vi "AES Encryption Example.vi"() -> ()   [LabVIEW 2016]
uses:
  <vilib>/Analysis/NI_AALBase.lvlib
panel:
  out "standard deviation":dbl format="%0.2f"
  out "mean":dbl format="%0.2f"
  out "String Length (Bytes)":i32
  out "Execution Time ms":dbl
  out "error out":errorcluster
  in  "Data to encrypt":string="Some crazy str data;\nI need to encrypt this with 256 bit encryption\nI hope <this> works (both ways)!"
  out "Plain Text":string
  out "CypheredText":string
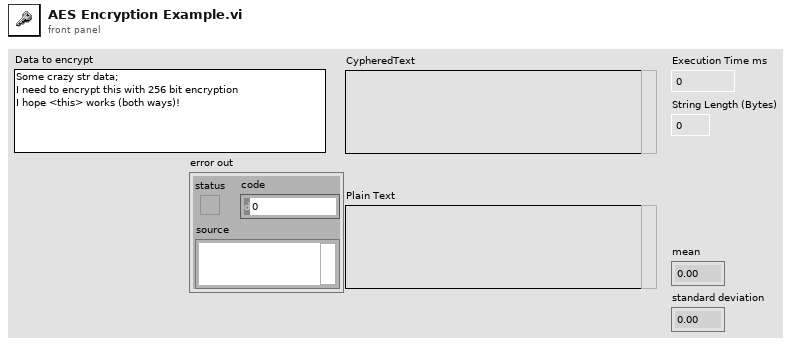
[diagram p1: front panel]
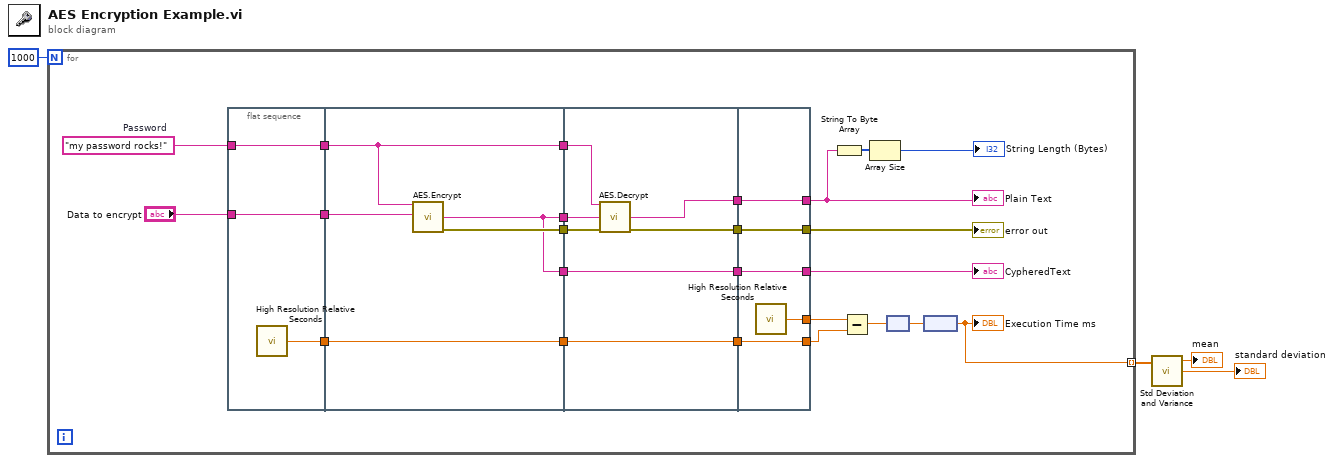
[diagram p0: block diagram]
diagram:
  n1 = for {
    N: 1000 -> [_]
    tunnel: [w5] -> w3 mode=indexing
    w16 = "my password rocks!"  # Password
    n2 = flat-sequence {
      tunnel: w16 -> [w30]
      tunnel: "Data to encrypt" -> [w31]
      tunnel: [w31] -> w28
      tunnel: [w30] -> w27
      tunnel: [w29] -> w26
      tunnel: [w33] -> w25
      tunnel: [w35] -> w24
      tunnel: w28 -> [w36]
      tunnel: w27 -> [w32]
      tunnel: [w34] -> w23
      tunnel: w26 -> [w34]
      tunnel: [w33] -> w22
      tunnel: [w32] -> w21
      tunnel: w25 -> [w39]
      tunnel: w24 -> [w42]
      tunnel: [w41] -> w20
      tunnel: [w43] -> w19
      tunnel: w23 -> [w43]
      tunnel: [w40] -> w18
      tunnel: w22 -> [w40]
      tunnel: w21 -> [w38]
      tunnel: [w37] -> w17
      tunnel: [w48] -> w11
      tunnel: w20 -> [w48]
      tunnel: [w47] -> w15
      tunnel: [w46] -> w14
      tunnel: w19 -> [w46]
      tunnel: [w45] -> w10
      tunnel: w18 -> [w45]
      tunnel: [w44] -> w8
      tunnel: w17 -> [w44]
      frame #0 {
        n3 = call <vilib>:"High Resolution Relative Seconds.vi"() -> ("relative seconds"=w29:dbl)
      }
      frame #1 {
        n4 = call <vilib>:"AES.Encrypt.vi"("Password"=w32, "PlainText"=w36) -> ("CypheredText"=w33:string, "error out"=w35:errorcluster)  [unwired: 12 in]
      }
      frame #2 {
        n5 = call <vilib>:"AES.Decrypt.vi"("Password"=w38, "EncryptedText"=w39, "error in"=w42) -> ("Plain Text"=w37:string, "error out"=w41:errorcluster)  [unwired: 11 in]
      }
      frame #3 {
        n6 = call <vilib>:"High Resolution Relative Seconds.vi"() -> ("relative seconds"=w47:dbl)
      }
    }
    n7 = String To Byte Array(string=w8) -> (unsigned byte array=w7:u8[])
    n8 = Subtract(x=w15, y=w14) -> (x-y=w13:dbl)
    n9 = Array Size(array=w7) -> (size(s)=→"String Length (Bytes)":i32)
    n10 = node(w13) -> (w12:dbl[unit])
    n11 = node(w12) -> (w5:dbl)
    "Execution Time ms" <- w5
    "Plain Text" <- w8
    "error out" <- w11
    "CypheredText" <- w10
  }
  n12 = call <vilib>:"Std Deviation and Variance.vi"("X"=w3) -> ("mean"=→"mean":dbl, "standard deviation"=→"standard deviation":dbl)  [unwired: 1 in, 1 out]
